vi "SetStreamingFilter.Do.vi"(8 "error in (no error)":errorcluster, 10 "State Variables":T1, 11 "gRPC Request":T13) -> (0 "error out":errorcluster, 2 "State Variables out":T1, 3 "gRPC Response":T14)   [LabVIEW 2025, in "bus_monitor_server_do.lvlib"]
uses:
  bus_monitor_server_do.lvlib
  Types/MainProcess.StateVariables.ctl
  Types/XNET.InitialSettings.ctl
  bus_monitor_server/RPC Messages/ni_bus_monitor_api_ConnectSettings.ctl
  bus_monitor_server/RPC Messages/ni_bus_monitor_api_CanMode.ctl
  bus_monitor_server/RPC Messages/ni_bus_monitor_api_Termination.ctl
  bus_monitor_server/RPC Messages/ni_bus_monitor_api_FdIsoMode.ctl
  bus_monitor_server/RPC Messages/ni_bus_monitor_api_FilterInfo.ctl
  bus_monitor_server/RPC Messages/ni_bus_monitor_api_DirectionFilter.ctl
  bus_monitor_server/RPC Messages/ni_bus_monitor_api_FrameFilter.ctl
  Types/StreamProcess.Refs.ctl
  Types/StreamProcess.VIRef.ctl
  bus_monitor_server/RPC Messages/ni_bus_monitor_api_Session.ctl
  bus_monitor_server/RPC Messages/ni_bus_monitor_api_SetStreamingFilterReply.ctl
  bus_monitor_server/RPC Messages/ni_bus_monitor_api_ErrorInfo.ctl
  bus_monitor_server/RPC Messages/ni_bus_monitor_api_SetStreamingFilterRequest.ctl
  bus_monitor_server/bus_monitor_server.lvlib
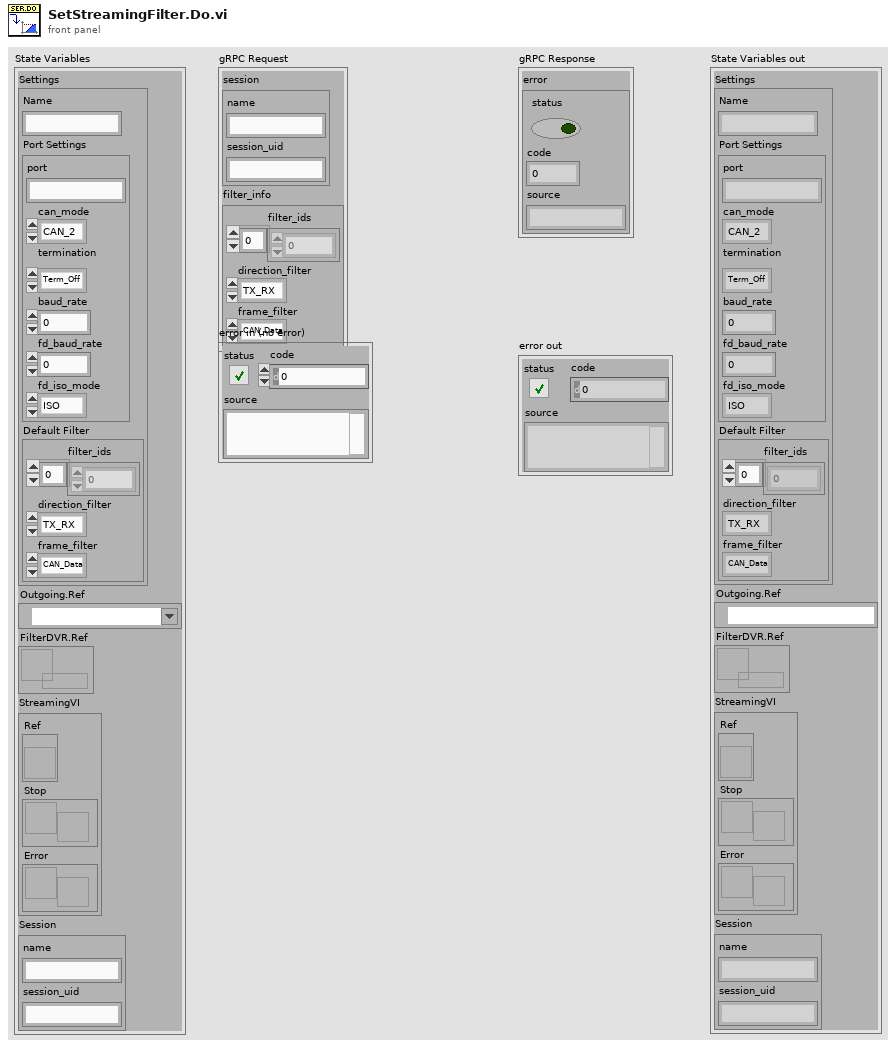
[diagram p1: front panel]
types:
  T1 = typedef "bus_monitor_server_do.lvlib/MainProcess.StateVariables.ctl" = cluster{"Settings":T2, "Outgoing.Ref":refnum<k21>, "FilterDVR.Ref":refnum<data-value>, "StreamingVI":T10, "Session":T12}
  T2 = typedef "bus_monitor_server_do.lvlib/XNET.InitialSettings.ctl" = cluster{"Name":string, "Port Settings":T3, "Default Filter":T7}
  T3 = typedef "bus_monitor_server.lvlib/ni_bus_monitor_api_ConnectSettings.ctl" = cluster{"port":string, "can_mode":T4, "termination":T5, "baud_rate":u64, "fd_baud_rate":u64, "fd_iso_mode":T6}
  T4 = typedef "bus_monitor_server.lvlib/ni_bus_monitor_api_CanMode.ctl" = enum32{"CAN_2", "CAN_FD", "CAN_FD_BRS"}
  T5 = typedef "bus_monitor_server.lvlib/ni_bus_monitor_api_Termination.ctl" = enum32{"Term_Off", "Term_On"}
  T6 = typedef "bus_monitor_server.lvlib/ni_bus_monitor_api_FdIsoMode.ctl" = enum32{"ISO", "Non_ISO", "ISO_Legacy"}
  T7 = typedef "bus_monitor_server.lvlib/ni_bus_monitor_api_FilterInfo.ctl" = cluster{"filter_ids":u32[], "direction_filter":T8, "frame_filter":T9}
  T8 = typedef "bus_monitor_server.lvlib/ni_bus_monitor_api_DirectionFilter.ctl" = enum32{"TX_RX", "RX", "TX"}
  T9 = typedef "bus_monitor_server.lvlib/ni_bus_monitor_api_FrameFilter.ctl" = enum32{"CAN_Data", "CAN_Remote", "CAN_Bus_Error", "CAN_2_Data", "CAN_FD_Data", "CAN_FD_BRS_Data", "J1939_Data", "Delay", "Log_Trigger", "Start_Trigger", "All"}
  T10 = typedef "bus_monitor_server_do.lvlib/StreamProcess.Refs.ctl" = cluster{"Ref":T11, "Stop":refnum<notifier>, "Error":refnum<notifier>}
  T11 = typedef "bus_monitor_server_do.lvlib/StreamProcess.VIRef.ctl" = refnum<vi>
  T12 = typedef "bus_monitor_server.lvlib/ni_bus_monitor_api_Session.ctl" = cluster{"name":string, "session_uid":string}
  T13 = typedef "bus_monitor_server.lvlib/ni_bus_monitor_api_SetStreamingFilterRequest.ctl" = cluster{"session":T12, "filter_info":T7}
  T14 = typedef "bus_monitor_server.lvlib/ni_bus_monitor_api_SetStreamingFilterReply.ctl" = cluster{"error":T15}
  T15 = typedef "bus_monitor_server.lvlib/ni_bus_monitor_api_ErrorInfo.ctl" = errorcluster
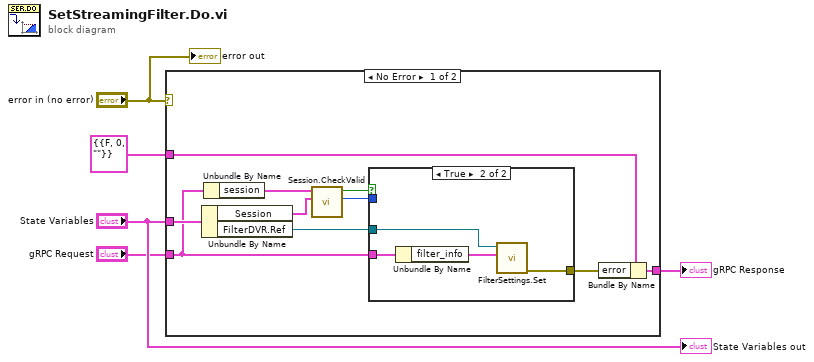
[diagram p0: block diagram]
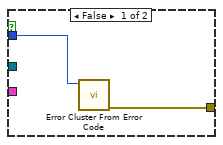
[diagram p2: hidden frame]
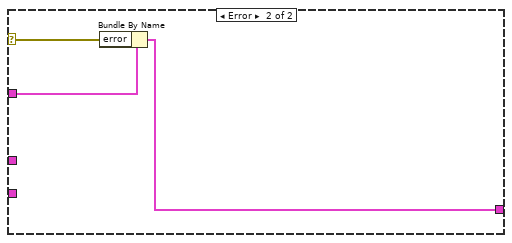
[diagram p3: hidden frame]
diagram:
  n1 = case shown="No Error" "error in (no error)" {
    selector: "error in (no error)" -> [_ w23]
    tunnel: "State Variables" -> [w15 _]
    tunnel: [w13 w22] -> w4
    tunnel: T14 {"error"={"status"=FALSE, "code"=0, "source"=""}} ("Message Data") -> [w12 w24]
    tunnel: "gRPC Request" -> [w10 _]
    frame No Error {
      n2 = Unbundle By Name(w15) -> ("Session"=w8:T12, "FilterDVR.Ref"=w14:refnum<data-value>)
      n3 = Unbundle By Name(w10) -> ("session"=w9:T12)
      n4 = call "Session.CheckValid.vi"("Cached Session"=w8, "requested session"=w9) -> ("Error Code"=w6:i32, "Valid?"=w7:bool)  [unwired: 8 in]
      n5 = case shown="True" w7 {
        tunnel: w10 -> [_ w20]
        tunnel: [w17 w21] -> w11
        tunnel: w14 -> [_ w18]
        tunnel: w6 -> [w16 _]
        frame False {
          n6 = call <vilib>:"Error Cluster From Error Code.vi"("error code (0)"=w16) -> ("error out"=w17:errorcluster)  [unwired: 8 in]
        }
        frame True {
          n7 = Unbundle By Name(w20) -> ("filter_info"=w19:T7)
          n8 = call "FilterSettings.Set.vi"("Filter"=w19, "FilterDVR.Ref"=w18) -> ("error out"=w21:errorcluster)  [unwired: 9 in]
        }
      }
      n9 = Bundle By Name(cluster=w12, "error"=w11) -> (w13:T14)
    }
    frame Error {
      n10 = Bundle By Name(cluster=w24, "error"=w23) -> (w22:T14)
    }
  }
  "gRPC Response" <- w4
  "State Variables out" <- "State Variables"
  "error out" <- "error in (no error)"
